vi "ExSubFullimage.vi"(2 "error in (no error)":errorcluster, 3 "Camera Handle":u32) -> (0 "error out":errorcluster, 1 "Camera Handle":u32)   [LabVIEW 2010]
uses:
  GlbCamHndls.vi
panel:
  # "ExSubFullImage:\nThis sub-vi gets the camera dimensions\nand picks/programs the full image."
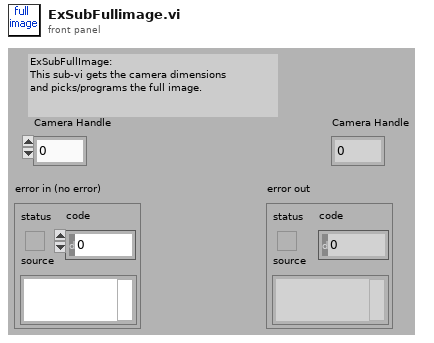
[diagram p1: front panel]
types:
  T1 = cluster{"X start":u32, "X end":u32, "X Binning/Grouping":u32, "Y start":u32, "Y end":u32, "Y Binning/Grouping":u32}
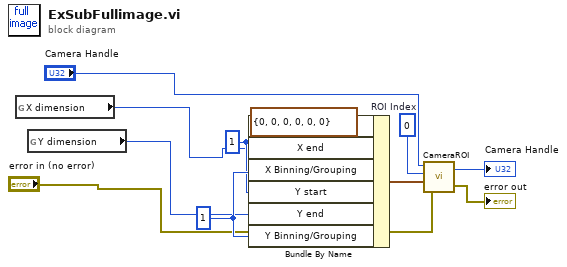
[diagram p0: block diagram]
diagram:
  w6 = u32 0  # ROI Index
  w9 = u32 1
  w5 = u32 1
  n1 = global read "GlbCamHndls.vi" "X dimension"() -> (w3:u32)
  n2 = global read "GlbCamHndls.vi" "Y dimension"() -> (w1:u32)
  n3 = Bundle By Name(cluster=T1 {"X start"=0, "X end"=0, "X Binning/Grouping"=0, "Y start"=0, "Y end"=0, "Y Binning/Grouping"=0} ("ROI Params"), "X start"=w5, "X end"=w3, "X Binning/Grouping"=w9, "Y start"=w5, "Y end"=w1, "Y Binning/Grouping"=w9) -> (w8:T1)
  n4 = call <userlib>:"CameraROI.vi"("error in"="error in (no error)", "ROI Params"=w8, "ROI Index"=w6, "Camera Handle"="Camera Handle") -> ("error out"=→"error out":errorcluster, "Camera Handle"=→"Camera Handle":u32)
